vi "RDS Router Subscribe.vi"(8 "error in (no error)":errorcluster, 10 "RDS Router Subscription":refnum<class "RDS Router Subscription.lvclass">, 11 "RDS Router Actor in":refnum<class "RDS Router Actor.lvclass">) -> (0 "error out":errorcluster, 3 "RDS Router Actor out":refnum<class "RDS Router Actor.lvclass">)   [LabVIEW 2015, in "RDS Abstracts.lvlib" / "RDS Router Actor.lvlib" / "RDS Router Actor.lvclass"]
uses:
  RDS Router Actor.lvclass
  RSD Subscription Class/RDS Router Subscription.lvclass
  RDS Router Actor.lvclass/RDS Router Actor.ctl
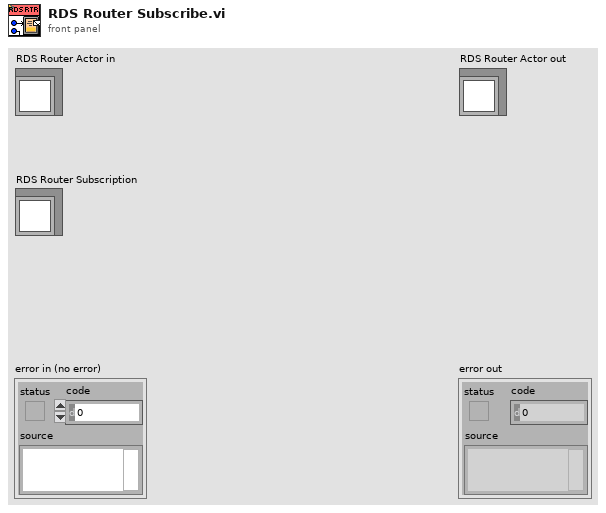
[diagram p1: front panel]
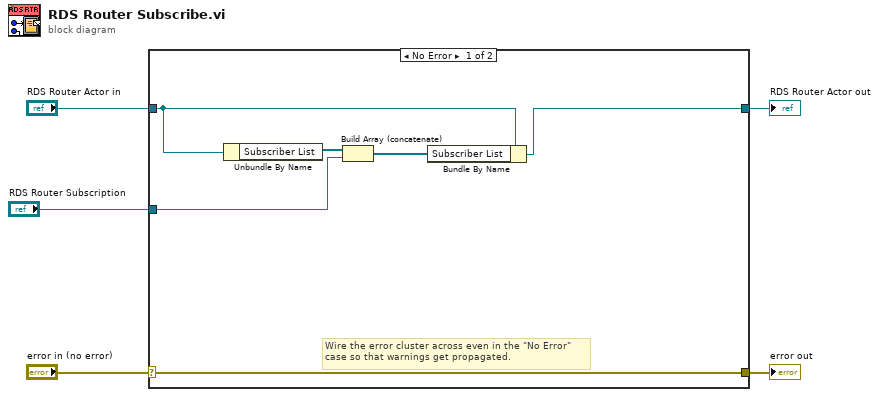
[diagram p0: block diagram]
diagram:
  n1 = case shown="No Error" "error in (no error)" {
    selector: "error in (no error)" -> [w11 w13]
    tunnel: [w11 w13] -> w4
    tunnel: [w6 w12] -> w2
    tunnel: "RDS Router Actor in" -> [w7 w12]
    tunnel: "RDS Router Subscription" -> [w9 _]
    frame No Error {
      # "Wire the error cluster across even in the \"No Error\"\ncase so that warnings get propagated."
      n2 = Unbundle By Name(w7) -> ("Subscriber List"=w10:refnum<class "RDS Router Subscription.lvclass">[])
      n3 = Build Array (concatenate)(w10, w9) -> (w8:refnum<class "RDS Router Subscription.lvclass">[])
      n4 = Bundle By Name(cluster=w7, "Subscriber List"=w8) -> (w6:refnum<class "RDS Router Actor.lvclass">)
    }
    frame Error {
    }
  }
  "error out" <- w4
  "RDS Router Actor out" <- w2
